vi "Datacluster_modify column.vi"(6 "tolerance":dbl=0.0005 format="%.3e", 7 "ascending":bool, 9 "Sort?":bool, 10 "Datasets to be processed":T3(array[cluster])=[{"String"="KR6_Rh3In3Ge4", "Boolean"=TRUE, "begin"=0, "length"=99, "y weight"=1.0}], 11 "data cluster":cluster{"all rows":dbl[][]}[](array[cluster])=[{"all rows"=[[292.0, 292.9164, 75.02219, 292.5198, 292.873, 0.08675399, 165.5123, 4.898979, 292.4821, 292.7706, 292.492, 292.5008, 293.2383, 292.873, 25.04327, 12.87815, 8.722502e-06, 147301.0, 0.0, 49.12202, 7.026817e-06], [292.0, 292.6799, 51.88008, 291.997, 292.6172, 0.1254523, 164.8345, 4.898979, 291.9992, 292.2308, 292.069, 291.9987, 292.9044, 292.6172, 16.68079, 8.502932, 7.87955e-06, 148972.5, 0.0, 52.73522, 7.82408e-06], [289.0, 289.5872, 53.36827, 288.998, 289.5262, 0.121954, 164.6135, 4.898979, 288.9966, 289.0375, 288.9818, 288.9977, 289.7039, 289.5262, 16.9019, 8.586199, 8.115929e-06, 149524.0, 0.0, 53.28857, 7.979706e-06], [286.0, 286.5259, 49.68945, 285.998, 286.4604, 0.130983, 164.4479, 4.898979, 285.9991, 285.8497, 285.9015, 285.9993, 286.5396, 286.4604, 16.3069, 8.351839, 7.550718e-06, 150070.2, 0.0, 49.26372, 7.019865e-06], [283.0, 283.4711, 53.72872, 283.0, 283.4105, 0.1211359, 164.3414, 4.898979, 282.9993, 282.7069, 282.8492, 283.0001, 283.3894, 283.4105, 16.49914, 8.324846, 8.321034e-06, 150632.6, 0.0, 53.01569, 7.9647e-06], [280.0, 280.4225, 55.74425, 280.001, 280.3641, 0.116756, 164.0834, 4.898979, 279.9989, 279.5874, 279.805, 279.9995, 280.2632, 280.3641, 16.65599, 8.355238, 8.692565e-06, 151182.8, 0.0, 57.0127, 8.356655e-06], [277.0, 277.4087, 53.59749, 277.0, 277.348, 0.1214324, 163.8697, 4.898979, 276.999, 276.4814, 276.7861, 277.0003, 277.1648, 277.348, 16.48811, 8.322479, 8.417088e-06, 151713.2, 0.0, 56.02918, 8.50766e-06], [274.0, 274.42, 54.6898, 274.001, 274.3605, 0.1190071, 163.7107, 4.898979, 273.9996, 273.4294, 273.7956, 274.0001, 274.1133, 274.3605, 16.45529, 8.266658, 8.774592e-06, 152257.0, 0.0, 55.53214, 8.58475e-06], [271.0, 271.4452, 55.7095, 271.001, 271.3868, 0.1168288, 163.585, 4.898979, 270.9994, 270.3922, 270.812, 270.9999, 271.0838, 271.3868, 16.27431, 8.125881, 8.904832e-06, 152814.4, 0.0, 56.2198, 8.635062e-06], [268.0, 268.4699, 56.23065, 268.001, 268.412, 0.115746, 163.4811, 4.898979, 267.9992, 267.3543, 267.8305, 267.9997, 268.0515, 268.412, 16.14259, 8.031859, 9.125312e-06, 153358.0, 0.0, 56.47631, 9.315139e-06], [265.0, 265.504, 56.7819, 265.0, 265.4467, 0.1146223, 163.391, 4.898979, 264.9995, 264.3426, 264.8619, 264.9997, 265.042, 265.4467, 16.08378, 7.981424, 9.334535e-06, 153898.2, 0.0, 56.33507, 9.071532e-06], [262.0, 262.5402, 56.3029, 261.999, 262.4824, 0.1155975, 163.3034, 4.898979, 261.9999, 261.3382, 261.8933, 262.0, 262.0429, 262.4824, 15.96119, 7.921869, 9.410211e-06, 154447.6, 0.0, 56.37045, 9.069828e-06], [259.0, 259.5962, 58.10709, 259.0, 259.5401, 0.1120083, 163.2193, 4.898979, 258.9994, 258.3609, 258.9463, 258.9997, 259.0668, 259.5401, 15.93857, 7.860623, 9.705625e-06, 154984.0, 0.0, 56.57644, 9.146704e-06], [256.0, 256.6687, 56.23365, 255.999, 256.6109, 0.1157399, 163.1493, 4.898979, 255.999, 255.398, 256.0085, 255.9989, 256.1162, 256.6109, 15.6581, 7.744409, 9.492895e-06, 155529.5, 0.0, 56.48109, 9.279682e-06], [253.0, 253.5733, 56.38813, 253.0, 253.53, 0.08656709, 163.0587, 4.242641, 252.9989, 252.4462, 253.0724, 252.9998, 252.9904, 253.53, 15.52846, 7.664103, 9.532705e-06, 156076.4, 0.0, 55.89689, 9.252784e-06], [250.0, 250.6412, 54.69462, 250.0, 250.5966, 0.08924747, 162.9786, 4.242641, 250.0002, 249.4823, 250.1305, 250.0004, 250.0376, 250.5966, 15.19496, 7.512066, 9.061377e-06, 156639.2, 0.0, 56.67262, 9.431853e-06], [247.0, 247.7008, 56.19418, 247.001, 247.6573, 0.08686587, 162.8957, 4.242641, 246.9987, 246.5324, 247.1849, 247.0003, 247.0917, 247.6573, 15.12285, 7.431846, 9.658179e-06, 157187.5, 0.0, 58.88652, 9.951588e-06], [244.0, 244.756, 57.27194, 243.999, 244.7134, 0.08523119, 162.8167, 4.242641, 243.9985, 243.5809, 244.2381, 243.9991, 244.1415, 244.7134, 15.06449, 7.372421, 1.015879e-05, 157736.6, 0.0, 57.34745, 9.89733e-06], [241.0, 241.8457, 56.35606, 240.999, 241.8024, 0.08661635, 162.7319, 4.242641, 240.9999, 240.6596, 241.3181, 240.9994, 241.2305, 241.8024, 14.76138, 7.218644, 1.001309e-05, 158281.2, 0.0, 55.59713, 9.467991e-06], [238.0, 238.9209, 56.78944, 238.0, 238.8779, 0.08595534, 162.6528, 4.242641, 237.9983, 237.7335, 238.3869, 237.9997, 238.3104, 238.8779, 14.65413, 7.147241, 9.925203e-06, 158821.8, 0.0, 57.4055, 9.991189e-06], [235.0, 235.8546, 58.50336, 235.0, 235.8233, 0.0625779, 162.5361, 3.674235, 234.9997, 234.8069, 235.452, 234.9992, 235.2407, 235.8233, 14.56547, 7.060409, 1.032292e-05, 159362.6, 0.0, 58.88609, 1.077016e-05], [232.0, 232.9135, 58.7887, 232.0, 232.8823, 0.06227416, 162.4497, 3.674235, 231.9992, 231.8697, 232.505, 232.0, 232.3093, 232.8823, 14.4148, 6.969601, 1.039831e-05, 159894.4, 0.0, 60.38943, 1.099243e-05], [229.0, 229.9683, 52.90027, 228.999, 229.9337, 0.06920602, 162.3651, 3.674235, 228.9996, 228.9262, 229.5497, 228.9995, 229.3795, 229.9337, 13.95679, 6.834046, 9.47672e-06, 160443.8, 0.0, 55.18934, 1.011709e-05], [226.0, 227.0314, 55.01033, 226.001, 226.9982, 0.06655145, 162.2802, 3.674235, 225.9986, 225.9999, 226.6072, 226.0003, 226.4574, 226.9982, 13.87658, 6.741458, 1.003314e-05, 160986.4, 0.0, 56.71966, 9.916942e-06], [223.0, 224.0942, 54.51703, 222.999, 224.0606, 0.06715364, 162.193, 3.674235, 222.9989, 223.0755, 223.6635, 222.999, 223.5397, 224.0606, 13.63051, 6.611919, 9.828761e-06, 161551.5, 0.0, 57.5095, 1.147469e-05], [220.0, 221.1488, 53.22712, 219.999, 221.1144, 0.06878105, 162.1079, 3.674235, 219.9987, 220.1357, 220.7061, 219.9996, 220.6128, 221.1144, 13.28219, 6.44084, 9.954398e-06, 162102.9, 0.0, 56.94044, 1.050179e-05], [217.0, 218.18, 55.6197, 217.0, 218.1471, 0.06582231, 162.0181, 3.674235, 216.9999, 217.1911, 217.7388, 216.9998, 217.6652, 218.1471, 13.33998, 6.426719, 1.030691e-05, 162650.0, 0.0, 54.95497, 1.056938e-05], [214.0, 215.2041, 52.74785, 214.001, 215.1694, 0.069406, 161.9245, 3.674235, 213.9993, 214.2305, 214.7574, 214.0001, 214.7119, 215.1694, 13.16094, 6.381908, 1.041787e-05, 163183.7, 0.0, 54.82949, 1.00501e-05], [211.0, 212.2438, 53.2594, 210.999, 212.2094, 0.06873936, 161.8459, 3.674235, 211.0002, 211.2871, 211.7895, 210.9995, 211.7758, 212.2094, 12.92852, 6.240668, 1.038931e-05, 163737.5, 0.0, 53.69054, 9.725446e-06], [208.0, 209.2728, 54.18705, 208.0, 209.239, 0.06756258, 161.7569, 3.674235, 207.9997, 208.341, 208.8189, 207.9994, 208.8287, 209.239, 12.96622, 6.244319, 1.030433e-05, 164296.5, 0.0, 51.99244, 9.937355e-06], [205.0, 206.3015, 47.85468, 204.999, 206.2633, 0.0765028, 161.669, 3.674235, 204.9996, 205.3777, 205.8335, 204.9997, 205.8839, 206.2633, 12.49721, 6.108157, 8.850608e-06, 164832.5, 0.0, 52.33099, 1.025279e-05], [202.0, 203.3115, 47.77909, 202.0, 203.2732, 0.07662382, 161.578, 3.674235, 201.9992, 202.4024, 202.836, 201.9998, 202.9163, 203.2732, 12.32563, 6.011273, 9.175306e-06, 165383.8, 0.0, 49.48042, 9.796374e-06], [199.0, 200.3016, 48.81196, 199.001, 200.2641, 0.07500245, 161.4837, 3.674235, 198.9994, 199.4091, 199.8188, 199.0009, 199.9294, 200.2641, 12.19196, 5.913105, 9.19541e-06, 165931.2, 0.0, 48.99235, 9.119814e-06], [196.0, 197.3124, 46.33101, 196.0, 197.2728, 0.07901871, 161.3904, 3.674235, 195.9999, 196.4343, 196.8208, 195.9996, 196.9654, 197.2728, 11.90443, 5.801792, 9.14851e-06, 166481.8, 0.0, 47.56836, 9.084771e-06], [193.0, 194.3294, 48.48906, 193.0, 194.2917, 0.07550192, 161.2938, 3.674235, 192.9996, 193.4505, 193.8166, 192.9997, 194.001, 194.2917, 11.49295, 5.526408, 9.320439e-06, 167039.8, 0.0, 49.01581, 9.34799e-06], [190.0, 191.3157, 47.75745, 189.999, 191.2773, 0.07665855, 161.2094, 3.674235, 190.0005, 190.4523, 190.7964, 189.9991, 191.0099, 191.2773, 11.31843, 5.442408, 9.51165e-06, 167586.2, 0.0, 47.72681, 9.290438e-06], [187.0, 188.2909, 46.66995, 186.998, 188.2517, 0.07844485, 161.1183, 3.674235, 186.9996, 187.4401, 187.7654, 187.0006, 188.0048, 188.2517, 11.22194, 5.408542, 9.210011e-06, 168125.0, 0.0, 47.7442, 9.335471e-06], [184.0, 185.2608, 45.59003, 184.0, 185.2207, 0.08030301, 161.02, 3.674235, 183.9996, 184.4185, 184.7246, 183.9997, 184.9949, 185.2207, 10.97692, 5.291597, 8.987941e-06, 168671.0, 0.0, 45.18603, 8.882518e-06], [181.0, 182.2488, 42.55964, 181.0, 182.2057, 0.08602087, 160.9233, 3.674235, 180.9996, 181.4114, 181.7032, 180.9994, 182.0001, 182.2057, 10.7433, 5.21988, 8.481294e-06, 169224.8, 0.0, 42.92117, 8.932989e-06], [178.0, 179.2327, 43.4817, 178.0, 179.1906, 0.08419672, 160.8244, 3.674235, 177.9992, 178.3866, 178.6756, 177.9989, 178.9857, 179.1906, 10.55317, 5.093926, 8.674955e-06, 169761.4, 0.0, 46.08075, 9.801831e-06], [175.0, 176.1988, 41.91763, 174.999, 176.1551, 0.08733836, 160.7272, 3.674235, 174.9992, 175.3492, 175.6323, 175.0005, 175.9594, 176.1551, 10.39018, 5.032765, 8.418331e-06, 170337.0, 0.0, 41.27729, 8.256854e-06], [172.0, 173.1462, 40.78401, 171.998, 173.1014, 0.08976599, 160.6309, 3.674235, 171.9994, 172.2934, 172.5681, 172.0007, 172.9165, 173.1014, 10.17369, 4.933174, 8.561175e-06, 170884.7, 0.0, 42.0311, 8.954053e-06], [169.0, 170.1156, 39.52542, 169.002, 170.0692, 0.09262438, 160.5319, 3.674235, 168.9985, 169.2597, 169.5281, 169.0004, 169.8935, 170.0692, 10.01111, 4.866947, 7.889127e-06, 171427.6, 0.0, 41.17875, 8.476864e-06], [166.0, 167.0848, 37.75683, 166.0, 167.0363, 0.09696304, 160.4351, 3.674235, 165.9992, 166.2177, 166.4835, 165.9991, 166.8676, 167.0363, 9.732579, 4.745978, 7.667965e-06, 171976.2, 0.0, 40.17138, 7.923543e-06], [163.0, 164.0348, 37.48756, 163.0, 163.986, 0.09765951, 160.3364, 3.674235, 162.9994, 163.1585, 163.4224, 162.9994, 163.8198, 163.986, 9.565177, 4.656068, 7.403833e-06, 172519.0, 0.0, 37.92251, 7.706918e-06], [160.0, 160.9789, 37.24322, 160.0, 160.9297, 0.09830023, 160.2345, 3.674235, 159.9997, 160.0851, 160.3523, 159.9997, 160.7607, 160.9297, 9.362346, 4.545693, 7.846706e-06, 173077.8, 0.0, 38.13007, 8.027448e-06], [157.0, 157.7978, 36.56221, 157.0, 157.7603, 0.07509838, 160.1422, 3.181981, 157.0001, 157.0355, 157.3161, 157.0001, 157.5547, 157.7603, 9.136679, 4.431653, 7.299468e-06, 173622.6, 0.0, 36.74182, 7.431135e-06], [154.0, 154.7562, 36.11287, 153.999, 154.7182, 0.0760328, 160.039, 3.181981, 154.0002, 153.9788, 154.2641, 153.9991, 154.5089, 154.7182, 8.931389, 4.324545, 7.829839e-06, 174165.6, 0.0, 37.11626, 7.907207e-06], [151.0, 151.7025, 35.56308, 151.001, 151.6639, 0.07720823, 159.94, 3.181981, 150.9997, 150.9063, 151.1997, 151.0003, 151.4478, 151.6639, 8.772177, 4.245581, 7.074522e-06, 174712.4, 0.0, 34.8322, 7.606191e-06], [148.0, 148.6425, 34.07633, 148.001, 148.6022, 0.08057683, 159.8368, 3.181981, 148.0007, 147.8203, 148.1272, 148.0007, 148.376, 148.6022, 8.538666, 4.143502, 7.012669e-06, 175270.5, 0.0, 35.5259, 7.773223e-06], [145.0, 145.6151, 32.94494, 145.0, 145.5734, 0.08334398, 159.7329, 3.181981, 144.9995, 144.7711, 145.0917, 145.0, 145.3362, 145.5734, 8.402115, 4.089585, 6.717016e-06, 175825.6, 0.0, 34.5873, 7.462285e-06], [142.0, 142.4503, 32.69128, 141.998, 142.4188, 0.062993, 159.6235, 2.755676, 141.9999, 141.7087, 142.045, 141.998, 142.1454, 142.4188, 8.112161, 3.93007, 6.970786e-06, 176365.9, 0.0, 33.20516, 7.879391e-06], [139.0, 139.3994, 31.76623, 139.001, 139.367, 0.06482741, 159.5169, 2.755676, 138.9981, 138.6308, 138.9849, 138.9994, 139.0777, 139.367, 7.985541, 3.877216, 6.982463e-06, 176903.8, 0.0, 32.45839, 6.596733e-06], [136.0, 136.3652, 31.01851, 135.998, 136.332, 0.0663901, 159.4101, 2.755676, 135.9989, 135.5674, 135.9417, 135.999, 136.0241, 136.332, 7.79429, 3.784086, 6.795836e-06, 177452.3, 0.0, 32.19581, 6.462182e-06], [133.0, 133.3502, 30.5601, 133.0, 133.3165, 0.06738596, 159.3015, 2.755676, 132.9992, 132.5206, 132.9147, 132.9999, 132.9898, 133.3165, 7.59515, 3.680558, 6.903421e-06, 178000.4, 0.0, 31.58324, 6.744551e-06], [130.0, 130.2115, 29.16558, 130.0, 130.185, 0.05295598, 159.122, 2.386485, 130.0005, 129.4585, 129.875, 129.9997, 129.8214, 130.185, 7.33831, 3.563506, 7.084772e-06, 178528.9, 0.0, 30.31422, 6.637657e-06], [127.0, 127.0902, 28.66261, 127.0, 127.07, 0.04041393, 159.0379, 2.066757, 126.9998, 126.3926, 126.8334, 126.9993, 126.6696, 127.07, 7.211448, 3.501876, 6.550803e-06, 179072.6, 0.0, 27.84635, 6.955272e-06], [124.0, 124.092, 28.58992, 124.0, 124.0717, 0.04051669, 158.9287, 2.066757, 124.0006, 123.3645, 123.8279, 123.9994, 123.6488, 124.0717, 7.012868, 3.390962, 7.173261e-06, 179624.9, 0.0, 28.22442, 4.92486e-06], [121.0, 121.0173, 26.81918, 120.999, 121.0011, 0.03239384, 158.8124, 1.789864, 120.9991, 120.3247, 120.8123, 120.9995, 120.5459, 121.0011, 6.797255, 3.304885, 4.45575e-06, 180140.8, 0.0, 29.19013, 5.915953e-06], [118.0, 117.9932, 25.80576, 117.999, 117.9764, 0.03366599, 158.6989, 1.789864, 117.9995, 117.2703, 117.781, 118.0, 117.4994, 117.9764, 6.568201, 3.195852, 5.482144e-06, 180683.1, 0.0, 27.08986, 6.913137e-06], [115.0, 115.0141, 25.65538, 114.998, 114.9971, 0.03386332, 158.5865, 1.789864, 115.0005, 114.2643, 114.7982, 114.9996, 114.497, 114.9971, 6.423356, 3.116589, 5.528924e-06, 181217.8, 0.0, 26.62919, 5.253105e-06], [112.0, 112.0203, 26.59349, 112.001, 112.004, 0.03266877, 158.4708, 1.789864, 111.9995, 111.2424, 111.7992, 111.9994, 111.4798, 112.004, 6.320665, 3.040642, 5.840544e-06, 181744.4, 0.0, 26.32533, 6.485414e-06], [109.0, 109.016, 25.89338, 109.0, 108.9992, 0.03355207, 158.3582, 1.789864, 109.0002, 108.2095, 108.7884, 108.9998, 108.4539, 108.9992, 6.13315, 2.948822, 4.976681e-06, 182293.6, 0.0, 25.56833, 6.586255e-06], [106.0, 106.0601, 24.74948, 105.999, 106.0426, 0.03510282, 158.2417, 1.789864, 106.0009, 105.2233, 105.8221, 105.9986, 105.4789, 106.0426, 5.82098, 2.795607, 5.520496e-06, 182820.9, 0.0, 25.1926, 5.082759e-06], [103.0, 103.1012, 23.47957, 102.999, 103.0827, 0.03700138, 158.1265, 1.789864, 102.9994, 102.2249, 102.852, 102.9995, 102.4926, 103.0827, 5.610787, 2.701479, 5.748678e-06, 183358.4, 0.0, 24.56658, 4.990891e-06], [100.0, 100.1194, 24.40213, 100.0, 100.1016, 0.03560248, 158.0093, 1.789864, 99.99963, 99.21942, 99.86005, 99.99973, 99.49659, 100.1016, 5.418124, 2.579388, 5.193695e-06, 183898.6, 0.0, 24.73305, 4.828259e-06], [97.0, 97.17382, 23.39176, 97.0015, 97.15525, 0.03714027, 157.8955, 1.789864, 96.99884, 96.25454, 96.90598, 96.99946, 96.54095, 97.15525, 5.252876, 2.504921, 5.62191e-06, 184439.7, 0.0, 23.73066, 5.229691e-06], [94.0, 94.20774, 23.22087, 94.0002, 94.18903, 0.0374136, 157.7782, 1.789864, 93.99808, 93.27039, 93.92858, 94.00004, 93.56826, 94.18903, 5.073145, 2.409457, 5.538685e-06, 184984.4, 0.0, 23.61211, 6.687232e-06], [91.0, 91.13359, 22.59694, 91.0003, 91.11917, 0.02883498, 157.6522, 1.550068, 91.0004, 90.31659, 90.91559, 90.9996, 90.54901, 91.11917, 4.827745, 2.285596, 4.255465e-06, 185533.6, 0.0, 21.92768, 5.296259e-06], [88.0, 88.18123, 22.48137, 87.9991, 88.16674, 0.02898322, 157.5325, 1.550068, 87.9996, 87.35154, 87.95371, 87.99927, 87.59355, 88.16674, 4.645815, 2.189353, 4.903361e-06, 186084.2, 0.0, 21.34062, 6.20428e-06], [85.0, 85.24232, 22.00163, 84.9979, 85.22751, 0.02961518, 157.4127, 1.550068, 85.00029, 84.40605, 85.0051, 84.99872, 84.65807, 85.22751, 4.439868, 2.085645, 3.898806e-06, 186641.8, 0.0, 20.03455, 4.048067e-06], [82.0, 82.2906, 20.26436, 82.0003, 82.27452, 0.0321541, 157.2935, 1.550068, 81.99943, 81.3944, 82.04882, 81.99944, 81.65225, 82.27452, 4.366601, 2.069786, 4.384861e-06, 187170.4, 0.0, 19.93068, 5.169709e-06], [79.0, 79.35992, 20.65986, 78.9998, 79.34415, 0.03153857, 157.175, 1.550068, 78.99976, 78.46501, 79.10271, 78.99972, 78.73799, 79.34415, 4.123809, 1.934396, 5.660535e-06, 187707.0, 0.0, 20.24228, 3.521332e-06], [76.0, 76.34799, 18.14755, 76.0001, 76.33453, 0.02692852, 157.0442, 1.342398, 75.9988, 75.52364, 76.14176, 76.00082, 75.74333, 76.33453, 3.879228, 1.836679, 5.277406e-06, 188227.8, 0.0, 18.3202, 4.280038e-06], [73.0, 73.40674, 18.83722, 72.9989, 73.39377, 0.02594261, 156.9286, 1.342398, 72.9991, 72.60294, 73.19315, 72.99918, 72.82951, 73.39377, 3.728216, 1.746902, 4.133453e-06, 188764.6, 0.0, 20.32012, 4.874801e-06], [70.0, 70.45695, 17.51673, 70.0003, 70.443, 0.02789829, 156.8115, 1.342398, 70.00086, 69.67221, 70.23128, 69.99956, 69.91183, 70.443, 3.505012, 1.644658, 3.415282e-06, 189312.8, 0.0, 18.10538, 3.636672e-06], [67.0, 67.51137, 17.06142, 66.9986, 67.49705, 0.0286428, 156.6926, 1.342398, 67.0003, 66.75251, 67.27265, 66.99976, 67.00556, 67.49705, 3.329935, 1.557489, 3.637388e-06, 189850.0, 0.0, 17.81273, 2.997229e-06], [64.0, 64.55299, 16.05667, 63.9994, 64.53777, 0.03043512, 156.572, 1.342398, 63.99965, 63.82388, 64.3001, 64.00019, 64.09199, 64.53777, 3.155975, 1.477454, 3.836114e-06, 190372.4, 0.0, 16.65761, 3.137167e-06], [61.0, 61.59684, 15.15327, 61.0012, 61.58071, 0.03224959, 156.4552, 1.342398, 61.00003, 60.89696, 61.32582, 60.99921, 61.18411, 61.58071, 2.932403, 1.370073, 2.715446e-06, 190890.4, 0.0, 15.46223, 4.794554e-06], [58.0, 58.6279, 14.0184, 58.0008, 58.61047, 0.03486038, 156.3434, 1.342398, 57.99915, 57.96364, 58.33762, 57.99934, 58.27135, 58.61047, 2.745862, 1.284894, 2.94282e-06, 191408.4, 0.0, 14.4151, 4.772166e-06], [55.0, 55.65962, 12.33515, 55.0029, 55.63981, 0.03961743, 156.2312, 1.342398, 54.99762, 55.02696, 55.34105, 55.0008, 55.36534, 55.63981, 2.519189, 1.185287, 3.164869e-06, 191919.5, 0.0, 12.86659, 1.828514e-06], [52.0, 52.69421, 11.21244, 51.999, 52.67242, 0.04358434, 156.12, 1.342398, 51.99888, 52.0955, 52.34609, 51.99949, 52.46542, 52.67242, 2.286444, 1.075562, 2.081657e-06, 192439.7, 0.0, 11.76603, 2.789106e-06], [49.0, 49.61418, 9.645293, 49.001, 49.59518, 0.03799937, 156.0042, 1.162551, 48.99919, 49.13845, 49.32293, 49.00038, 49.4487, 49.59518, 2.049105, 0.9693383, 2.419945e-06, 192925.6, 0.0, 10.21014, 2.551699e-06], [46.0, 46.64398, 8.849838, 46.0014, 46.62327, 0.04141489, 155.8991, 1.162551, 45.99971, 46.20159, 46.31906, 45.99925, 46.54721, 46.62327, 1.829977, 0.8624549, 2.062263e-06, 193484.8, 0.0, 8.642792, 8.766135e-07], [43.0, 43.63805, 8.111564, 43.0, 43.61546, 0.04518427, 155.7963, 1.162551, 43.00087, 43.23263, 43.28277, 42.99939, 43.6105, 43.61546, 1.669476, 0.7863123, 2.202847e-06, 194031.9, 0.0, 8.304894, 2.187056e-06], [40.0, 40.60721, 7.850611, 39.9976, 40.58387, 0.04668618, 155.6928, 1.162551, 39.99903, 40.24392, 40.22946, 39.99922, 40.64502, 40.58387, 1.579687, 0.7417823, 1.934699e-06, 194511.3, 0.0, 7.823251, 1.052641e-06], [37.0, 37.55588, 7.570818, 37.0021, 37.53168, 0.04841156, 155.5887, 1.162551, 36.99997, 37.23081, 37.15568, 36.99985, 37.65521, 37.53168, 1.491856, 0.6986331, 1.616464e-06, 195029.6, 0.0, 7.701154, 1.426829e-06], [34.0, 34.39013, 7.129456, 34.002, 34.37085, 0.03855642, 155.4653, 1.006799, 34.00288, 34.19961, 34.07078, 33.99971, 34.53824, 34.37085, 1.389701, 0.6498903, 1.456064e-06, 195501.9, 0.0, 7.197325, 1.830936e-06], [31.0, 31.3295, 6.959681, 30.9971, 31.30975, 0.03949697, 155.3693, 1.006799, 31.00027, 31.15947, 30.98673, 30.99905, 31.52198, 31.30975, 1.305866, 0.6077944, 1.746532e-06, 195974.6, 0.0, 6.855044, 1.3535e-07], [28.0, 28.257, 6.444445, 28.0083, 28.23568, 0.04265477, 155.2754, 1.006799, 27.99751, 28.08427, 27.88122, 28.00025, 28.48138, 28.23568, 1.20443, 0.5603139, 1.207888e-06, 196438.7, 0.0, 6.465166, 2.29124e-06], [25.0, 25.1858, 5.908139, 25.0055, 25.16253, 0.04652672, 155.1906, 1.006799, 25.00147, 24.99086, 24.77406, 24.99832, 25.42586, 25.16253, 1.084087, 0.5032175, 9.614257e-07, 196931.6, 0.0, 5.92471, -5.51895e-08], [22.0, 22.16916, 5.305623, 21.9854, 22.14325, 0.05181037, 155.1142, 1.006799, 22.00671, 21.91764, 21.70696, 21.99982, 22.40575, 22.14325, 0.959603, 0.4446781, 7.916026e-07, 197380.4, 0.0, 5.277611, 2.768679e-07], [19.0, 19.30572, 4.637635, 18.9844, 19.27608, 0.05927295, 155.0499, 1.006799, 18.99661, 18.95241, 18.76765, 19.00061, 19.52011, 19.27608, 0.8426237, 0.390679, 5.587576e-07, 197860.4, 0.0, 4.670142, -7.621961e-08], [16.0, 16.50024, 3.972702, 16.0034, 16.46565, 0.06919378, 154.9962, 1.006799, 15.99681, 16.00464, 15.86607, 15.99389, 16.67341, 16.46565, 0.7071578, 0.3270905, 3.955843e-07, 198345.2, 0.0, 3.981336, -9.093087e-09], [13.0, 13.71888, 3.255681, 13.0265, 13.67666, 0.08443282, 154.9529, 1.006799, 12.99021, 12.98951, 12.9155, 12.99523, 13.83511, 13.67666, 0.5650661, 0.2606204, 4.899574e-08, 199058.5, 0.0, 3.267024, -3.089664e-07], [10.0, 11.02144, 2.634719, 9.9178, 10.96927, 0.1043323, 154.9244, 1.006799, 9.979209, 9.944225, 9.937939, 9.981572, 11.07989, 10.96927, 0.4191188, 0.1915213, 3.509129e-08, 199788.6, 0.0, 2.637912, 3.892924e-07], [7.0, 8.207977, 2.280254, 7.0263, 8.162771, 0.09041306, 154.877, 0.8719131, 6.996675, 6.899136, 6.944581, 6.995916, 8.207738, 8.162771, 0.272072, 0.1212537, 1.590448e-07, 200474.8, 0.0, 2.226699, -2.06841e-07], [4.0, 6.17061, 6.914511, 3.9852, 6.155702, 0.02981624, 154.8519, 0.8719131, 4.007358, 3.946248, 3.912001, 4.007225, 6.219766, 6.155702, 0.1566822, 0.06587024, 3.496313e-07, 201190.7, 0.0, 6.388795, -3.268214e-08], [2.0, 3.439481, -0.8426919, 2.2818, 3.470062, -0.06116255, 154.8119, 0.4359565, 2.275721, 2.314741, 2.136495, 2.275818, 3.587147, 3.470062, 0.06999886, 0.02771, -3.623877e-09, 201712.2, 0.0, -0.8426919, -3.623877e-09]]}]) -> (3 "data cluster out":cluster{"all rows":dbl[][]}[](array[cluster])=[{"all rows"=[[292.0, 292.9164, 75.02219, 292.5198, 292.873, 0.08675399, 165.5123, 4.898979, 292.4821, 292.7706, 292.492, 292.5008, 293.2383, 292.873, 25.04327, 12.87815, 8.722502e-06, 147301.0, 0.0, 49.12202, 7.026817e-06], [292.0, 292.6799, 51.88008, 291.997, 292.6172, 0.1254523, 164.8345, 4.898979, 291.9992, 292.2308, 292.069, 291.9987, 292.9044, 292.6172, 16.68079, 8.502932, 7.87955e-06, 148972.5, 0.0, 52.73522, 7.82408e-06], [289.0, 289.5872, 53.36827, 288.998, 289.5262, 0.121954, 164.6135, 4.898979, 288.9966, 289.0375, 288.9818, 288.9977, 289.7039, 289.5262, 16.9019, 8.586199, 8.115929e-06, 149524.0, 0.0, 53.28857, 7.979706e-06], [286.0, 286.5259, 49.68945, 285.998, 286.4604, 0.130983, 164.4479, 4.898979, 285.9991, 285.8497, 285.9015, 285.9993, 286.5396, 286.4604, 16.3069, 8.351839, 7.550718e-06, 150070.2, 0.0, 49.26372, 7.019865e-06], [283.0, 283.4711, 53.72872, 283.0, 283.4105, 0.1211359, 164.3414, 4.898979, 282.9993, 282.7069, 282.8492, 283.0001, 283.3894, 283.4105, 16.49914, 8.324846, 8.321034e-06, 150632.6, 0.0, 53.01569, 7.9647e-06], [280.0, 280.4225, 55.74425, 280.001, 280.3641, 0.116756, 164.0834, 4.898979, 279.9989, 279.5874, 279.805, 279.9995, 280.2632, 280.3641, 16.65599, 8.355238, 8.692565e-06, 151182.8, 0.0, 57.0127, 8.356655e-06], [277.0, 277.4087, 53.59749, 277.0, 277.348, 0.1214324, 163.8697, 4.898979, 276.999, 276.4814, 276.7861, 277.0003, 277.1648, 277.348, 16.48811, 8.322479, 8.417088e-06, 151713.2, 0.0, 56.02918, 8.50766e-06], [274.0, 274.42, 54.6898, 274.001, 274.3605, 0.1190071, 163.7107, 4.898979, 273.9996, 273.4294, 273.7956, 274.0001, 274.1133, 274.3605, 16.45529, 8.266658, 8.774592e-06, 152257.0, 0.0, 55.53214, 8.58475e-06], [271.0, 271.4452, 55.7095, 271.001, 271.3868, 0.1168288, 163.585, 4.898979, 270.9994, 270.3922, 270.812, 270.9999, 271.0838, 271.3868, 16.27431, 8.125881, 8.904832e-06, 152814.4, 0.0, 56.2198, 8.635062e-06], [268.0, 268.4699, 56.23065, 268.001, 268.412, 0.115746, 163.4811, 4.898979, 267.9992, 267.3543, 267.8305, 267.9997, 268.0515, 268.412, 16.14259, 8.031859, 9.125312e-06, 153358.0, 0.0, 56.47631, 9.315139e-06], [265.0, 265.504, 56.7819, 265.0, 265.4467, 0.1146223, 163.391, 4.898979, 264.9995, 264.3426, 264.8619, 264.9997, 265.042, 265.4467, 16.08378, 7.981424, 9.334535e-06, 153898.2, 0.0, 56.33507, 9.071532e-06], [262.0, 262.5402, 56.3029, 261.999, 262.4824, 0.1155975, 163.3034, 4.898979, 261.9999, 261.3382, 261.8933, 262.0, 262.0429, 262.4824, 15.96119, 7.921869, 9.410211e-06, 154447.6, 0.0, 56.37045, 9.069828e-06], [259.0, 259.5962, 58.10709, 259.0, 259.5401, 0.1120083, 163.2193, 4.898979, 258.9994, 258.3609, 258.9463, 258.9997, 259.0668, 259.5401, 15.93857, 7.860623, 9.705625e-06, 154984.0, 0.0, 56.57644, 9.146704e-06], [256.0, 256.6687, 56.23365, 255.999, 256.6109, 0.1157399, 163.1493, 4.898979, 255.999, 255.398, 256.0085, 255.9989, 256.1162, 256.6109, 15.6581, 7.744409, 9.492895e-06, 155529.5, 0.0, 56.48109, 9.279682e-06], [253.0, 253.5733, 56.38813, 253.0, 253.53, 0.08656709, 163.0587, 4.242641, 252.9989, 252.4462, 253.0724, 252.9998, 252.9904, 253.53, 15.52846, 7.664103, 9.532705e-06, 156076.4, 0.0, 55.89689, 9.252784e-06], [250.0, 250.6412, 54.69462, 250.0, 250.5966, 0.08924747, 162.9786, 4.242641, 250.0002, 249.4823, 250.1305, 250.0004, 250.0376, 250.5966, 15.19496, 7.512066, 9.061377e-06, 156639.2, 0.0, 56.67262, 9.431853e-06], [247.0, 247.7008, 56.19418, 247.001, 247.6573, 0.08686587, 162.8957, 4.242641, 246.9987, 246.5324, 247.1849, 247.0003, 247.0917, 247.6573, 15.12285, 7.431846, 9.658179e-06, 157187.5, 0.0, 58.88652, 9.951588e-06], [244.0, 244.756, 57.27194, 243.999, 244.7134, 0.08523119, 162.8167, 4.242641, 243.9985, 243.5809, 244.2381, 243.9991, 244.1415, 244.7134, 15.06449, 7.372421, 1.015879e-05, 157736.6, 0.0, 57.34745, 9.89733e-06], [241.0, 241.8457, 56.35606, 240.999, 241.8024, 0.08661635, 162.7319, 4.242641, 240.9999, 240.6596, 241.3181, 240.9994, 241.2305, 241.8024, 14.76138, 7.218644, 1.001309e-05, 158281.2, 0.0, 55.59713, 9.467991e-06], [238.0, 238.9209, 56.78944, 238.0, 238.8779, 0.08595534, 162.6528, 4.242641, 237.9983, 237.7335, 238.3869, 237.9997, 238.3104, 238.8779, 14.65413, 7.147241, 9.925203e-06, 158821.8, 0.0, 57.4055, 9.991189e-06], [235.0, 235.8546, 58.50336, 235.0, 235.8233, 0.0625779, 162.5361, 3.674235, 234.9997, 234.8069, 235.452, 234.9992, 235.2407, 235.8233, 14.56547, 7.060409, 1.032292e-05, 159362.6, 0.0, 58.88609, 1.077016e-05], [232.0, 232.9135, 58.7887, 232.0, 232.8823, 0.06227416, 162.4497, 3.674235, 231.9992, 231.8697, 232.505, 232.0, 232.3093, 232.8823, 14.4148, 6.969601, 1.039831e-05, 159894.4, 0.0, 60.38943, 1.099243e-05], [229.0, 229.9683, 52.90027, 228.999, 229.9337, 0.06920602, 162.3651, 3.674235, 228.9996, 228.9262, 229.5497, 228.9995, 229.3795, 229.9337, 13.95679, 6.834046, 9.47672e-06, 160443.8, 0.0, 55.18934, 1.011709e-05], [226.0, 227.0314, 55.01033, 226.001, 226.9982, 0.06655145, 162.2802, 3.674235, 225.9986, 225.9999, 226.6072, 226.0003, 226.4574, 226.9982, 13.87658, 6.741458, 1.003314e-05, 160986.4, 0.0, 56.71966, 9.916942e-06], [223.0, 224.0942, 54.51703, 222.999, 224.0606, 0.06715364, 162.193, 3.674235, 222.9989, 223.0755, 223.6635, 222.999, 223.5397, 224.0606, 13.63051, 6.611919, 9.828761e-06, 161551.5, 0.0, 57.5095, 1.147469e-05], [220.0, 221.1488, 53.22712, 219.999, 221.1144, 0.06878105, 162.1079, 3.674235, 219.9987, 220.1357, 220.7061, 219.9996, 220.6128, 221.1144, 13.28219, 6.44084, 9.954398e-06, 162102.9, 0.0, 56.94044, 1.050179e-05], [217.0, 218.18, 55.6197, 217.0, 218.1471, 0.06582231, 162.0181, 3.674235, 216.9999, 217.1911, 217.7388, 216.9998, 217.6652, 218.1471, 13.33998, 6.426719, 1.030691e-05, 162650.0, 0.0, 54.95497, 1.056938e-05], [214.0, 215.2041, 52.74785, 214.001, 215.1694, 0.069406, 161.9245, 3.674235, 213.9993, 214.2305, 214.7574, 214.0001, 214.7119, 215.1694, 13.16094, 6.381908, 1.041787e-05, 163183.7, 0.0, 54.82949, 1.00501e-05], [211.0, 212.2438, 53.2594, 210.999, 212.2094, 0.06873936, 161.8459, 3.674235, 211.0002, 211.2871, 211.7895, 210.9995, 211.7758, 212.2094, 12.92852, 6.240668, 1.038931e-05, 163737.5, 0.0, 53.69054, 9.725446e-06], [208.0, 209.2728, 54.18705, 208.0, 209.239, 0.06756258, 161.7569, 3.674235, 207.9997, 208.341, 208.8189, 207.9994, 208.8287, 209.239, 12.96622, 6.244319, 1.030433e-05, 164296.5, 0.0, 51.99244, 9.937355e-06], [205.0, 206.3015, 47.85468, 204.999, 206.2633, 0.0765028, 161.669, 3.674235, 204.9996, 205.3777, 205.8335, 204.9997, 205.8839, 206.2633, 12.49721, 6.108157, 8.850608e-06, 164832.5, 0.0, 52.33099, 1.025279e-05], [202.0, 203.3115, 47.77909, 202.0, 203.2732, 0.07662382, 161.578, 3.674235, 201.9992, 202.4024, 202.836, 201.9998, 202.9163, 203.2732, 12.32563, 6.011273, 9.175306e-06, 165383.8, 0.0, 49.48042, 9.796374e-06], [199.0, 200.3016, 48.81196, 199.001, 200.2641, 0.07500245, 161.4837, 3.674235, 198.9994, 199.4091, 199.8188, 199.0009, 199.9294, 200.2641, 12.19196, 5.913105, 9.19541e-06, 165931.2, 0.0, 48.99235, 9.119814e-06], [196.0, 197.3124, 46.33101, 196.0, 197.2728, 0.07901871, 161.3904, 3.674235, 195.9999, 196.4343, 196.8208, 195.9996, 196.9654, 197.2728, 11.90443, 5.801792, 9.14851e-06, 166481.8, 0.0, 47.56836, 9.084771e-06], [193.0, 194.3294, 48.48906, 193.0, 194.2917, 0.07550192, 161.2938, 3.674235, 192.9996, 193.4505, 193.8166, 192.9997, 194.001, 194.2917, 11.49295, 5.526408, 9.320439e-06, 167039.8, 0.0, 49.01581, 9.34799e-06], [190.0, 191.3157, 47.75745, 189.999, 191.2773, 0.07665855, 161.2094, 3.674235, 190.0005, 190.4523, 190.7964, 189.9991, 191.0099, 191.2773, 11.31843, 5.442408, 9.51165e-06, 167586.2, 0.0, 47.72681, 9.290438e-06], [187.0, 188.2909, 46.66995, 186.998, 188.2517, 0.07844485, 161.1183, 3.674235, 186.9996, 187.4401, 187.7654, 187.0006, 188.0048, 188.2517, 11.22194, 5.408542, 9.210011e-06, 168125.0, 0.0, 47.7442, 9.335471e-06], [184.0, 185.2608, 45.59003, 184.0, 185.2207, 0.08030301, 161.02, 3.674235, 183.9996, 184.4185, 184.7246, 183.9997, 184.9949, 185.2207, 10.97692, 5.291597, 8.987941e-06, 168671.0, 0.0, 45.18603, 8.882518e-06], [181.0, 182.2488, 42.55964, 181.0, 182.2057, 0.08602087, 160.9233, 3.674235, 180.9996, 181.4114, 181.7032, 180.9994, 182.0001, 182.2057, 10.7433, 5.21988, 8.481294e-06, 169224.8, 0.0, 42.92117, 8.932989e-06], [178.0, 179.2327, 43.4817, 178.0, 179.1906, 0.08419672, 160.8244, 3.674235, 177.9992, 178.3866, 178.6756, 177.9989, 178.9857, 179.1906, 10.55317, 5.093926, 8.674955e-06, 169761.4, 0.0, 46.08075, 9.801831e-06], [175.0, 176.1988, 41.91763, 174.999, 176.1551, 0.08733836, 160.7272, 3.674235, 174.9992, 175.3492, 175.6323, 175.0005, 175.9594, 176.1551, 10.39018, 5.032765, 8.418331e-06, 170337.0, 0.0, 41.27729, 8.256854e-06], [172.0, 173.1462, 40.78401, 171.998, 173.1014, 0.08976599, 160.6309, 3.674235, 171.9994, 172.2934, 172.5681, 172.0007, 172.9165, 173.1014, 10.17369, 4.933174, 8.561175e-06, 170884.7, 0.0, 42.0311, 8.954053e-06], [169.0, 170.1156, 39.52542, 169.002, 170.0692, 0.09262438, 160.5319, 3.674235, 168.9985, 169.2597, 169.5281, 169.0004, 169.8935, 170.0692, 10.01111, 4.866947, 7.889127e-06, 171427.6, 0.0, 41.17875, 8.476864e-06], [166.0, 167.0848, 37.75683, 166.0, 167.0363, 0.09696304, 160.4351, 3.674235, 165.9992, 166.2177, 166.4835, 165.9991, 166.8676, 167.0363, 9.732579, 4.745978, 7.667965e-06, 171976.2, 0.0, 40.17138, 7.923543e-06], [163.0, 164.0348, 37.48756, 163.0, 163.986, 0.09765951, 160.3364, 3.674235, 162.9994, 163.1585, 163.4224, 162.9994, 163.8198, 163.986, 9.565177, 4.656068, 7.403833e-06, 172519.0, 0.0, 37.92251, 7.706918e-06], [160.0, 160.9789, 37.24322, 160.0, 160.9297, 0.09830023, 160.2345, 3.674235, 159.9997, 160.0851, 160.3523, 159.9997, 160.7607, 160.9297, 9.362346, 4.545693, 7.846706e-06, 173077.8, 0.0, 38.13007, 8.027448e-06], [157.0, 157.7978, 36.56221, 157.0, 157.7603, 0.07509838, 160.1422, 3.181981, 157.0001, 157.0355, 157.3161, 157.0001, 157.5547, 157.7603, 9.136679, 4.431653, 7.299468e-06, 173622.6, 0.0, 36.74182, 7.431135e-06], [154.0, 154.7562, 36.11287, 153.999, 154.7182, 0.0760328, 160.039, 3.181981, 154.0002, 153.9788, 154.2641, 153.9991, 154.5089, 154.7182, 8.931389, 4.324545, 7.829839e-06, 174165.6, 0.0, 37.11626, 7.907207e-06], [151.0, 151.7025, 35.56308, 151.001, 151.6639, 0.07720823, 159.94, 3.181981, 150.9997, 150.9063, 151.1997, 151.0003, 151.4478, 151.6639, 8.772177, 4.245581, 7.074522e-06, 174712.4, 0.0, 34.8322, 7.606191e-06], [148.0, 148.6425, 34.07633, 148.001, 148.6022, 0.08057683, 159.8368, 3.181981, 148.0007, 147.8203, 148.1272, 148.0007, 148.376, 148.6022, 8.538666, 4.143502, 7.012669e-06, 175270.5, 0.0, 35.5259, 7.773223e-06], [145.0, 145.6151, 32.94494, 145.0, 145.5734, 0.08334398, 159.7329, 3.181981, 144.9995, 144.7711, 145.0917, 145.0, 145.3362, 145.5734, 8.402115, 4.089585, 6.717016e-06, 175825.6, 0.0, 34.5873, 7.462285e-06], [142.0, 142.4503, 32.69128, 141.998, 142.4188, 0.062993, 159.6235, 2.755676, 141.9999, 141.7087, 142.045, 141.998, 142.1454, 142.4188, 8.112161, 3.93007, 6.970786e-06, 176365.9, 0.0, 33.20516, 7.879391e-06], [139.0, 139.3994, 31.76623, 139.001, 139.367, 0.06482741, 159.5169, 2.755676, 138.9981, 138.6308, 138.9849, 138.9994, 139.0777, 139.367, 7.985541, 3.877216, 6.982463e-06, 176903.8, 0.0, 32.45839, 6.596733e-06], [136.0, 136.3652, 31.01851, 135.998, 136.332, 0.0663901, 159.4101, 2.755676, 135.9989, 135.5674, 135.9417, 135.999, 136.0241, 136.332, 7.79429, 3.784086, 6.795836e-06, 177452.3, 0.0, 32.19581, 6.462182e-06], [133.0, 133.3502, 30.5601, 133.0, 133.3165, 0.06738596, 159.3015, 2.755676, 132.9992, 132.5206, 132.9147, 132.9999, 132.9898, 133.3165, 7.59515, 3.680558, 6.903421e-06, 178000.4, 0.0, 31.58324, 6.744551e-06], [130.0, 130.2115, 29.16558, 130.0, 130.185, 0.05295598, 159.122, 2.386485, 130.0005, 129.4585, 129.875, 129.9997, 129.8214, 130.185, 7.33831, 3.563506, 7.084772e-06, 178528.9, 0.0, 30.31422, 6.637657e-06], [127.0, 127.0902, 28.66261, 127.0, 127.07, 0.04041393, 159.0379, 2.066757, 126.9998, 126.3926, 126.8334, 126.9993, 126.6696, 127.07, 7.211448, 3.501876, 6.550803e-06, 179072.6, 0.0, 27.84635, 6.955272e-06], [124.0, 124.092, 28.58992, 124.0, 124.0717, 0.04051669, 158.9287, 2.066757, 124.0006, 123.3645, 123.8279, 123.9994, 123.6488, 124.0717, 7.012868, 3.390962, 7.173261e-06, 179624.9, 0.0, 28.22442, 4.92486e-06], [121.0, 121.0173, 26.81918, 120.999, 121.0011, 0.03239384, 158.8124, 1.789864, 120.9991, 120.3247, 120.8123, 120.9995, 120.5459, 121.0011, 6.797255, 3.304885, 4.45575e-06, 180140.8, 0.0, 29.19013, 5.915953e-06], [118.0, 117.9932, 25.80576, 117.999, 117.9764, 0.03366599, 158.6989, 1.789864, 117.9995, 117.2703, 117.781, 118.0, 117.4994, 117.9764, 6.568201, 3.195852, 5.482144e-06, 180683.1, 0.0, 27.08986, 6.913137e-06], [115.0, 115.0141, 25.65538, 114.998, 114.9971, 0.03386332, 158.5865, 1.789864, 115.0005, 114.2643, 114.7982, 114.9996, 114.497, 114.9971, 6.423356, 3.116589, 5.528924e-06, 181217.8, 0.0, 26.62919, 5.253105e-06], [112.0, 112.0203, 26.59349, 112.001, 112.004, 0.03266877, 158.4708, 1.789864, 111.9995, 111.2424, 111.7992, 111.9994, 111.4798, 112.004, 6.320665, 3.040642, 5.840544e-06, 181744.4, 0.0, 26.32533, 6.485414e-06], [109.0, 109.016, 25.89338, 109.0, 108.9992, 0.03355207, 158.3582, 1.789864, 109.0002, 108.2095, 108.7884, 108.9998, 108.4539, 108.9992, 6.13315, 2.948822, 4.976681e-06, 182293.6, 0.0, 25.56833, 6.586255e-06], [106.0, 106.0601, 24.74948, 105.999, 106.0426, 0.03510282, 158.2417, 1.789864, 106.0009, 105.2233, 105.8221, 105.9986, 105.4789, 106.0426, 5.82098, 2.795607, 5.520496e-06, 182820.9, 0.0, 25.1926, 5.082759e-06], [103.0, 103.1012, 23.47957, 102.999, 103.0827, 0.03700138, 158.1265, 1.789864, 102.9994, 102.2249, 102.852, 102.9995, 102.4926, 103.0827, 5.610787, 2.701479, 5.748678e-06, 183358.4, 0.0, 24.56658, 4.990891e-06], [100.0, 100.1194, 24.40213, 100.0, 100.1016, 0.03560248, 158.0093, 1.789864, 99.99963, 99.21942, 99.86005, 99.99973, 99.49659, 100.1016, 5.418124, 2.579388, 5.193695e-06, 183898.6, 0.0, 24.73305, 4.828259e-06], [97.0, 97.17382, 23.39176, 97.0015, 97.15525, 0.03714027, 157.8955, 1.789864, 96.99884, 96.25454, 96.90598, 96.99946, 96.54095, 97.15525, 5.252876, 2.504921, 5.62191e-06, 184439.7, 0.0, 23.73066, 5.229691e-06], [94.0, 94.20774, 23.22087, 94.0002, 94.18903, 0.0374136, 157.7782, 1.789864, 93.99808, 93.27039, 93.92858, 94.00004, 93.56826, 94.18903, 5.073145, 2.409457, 5.538685e-06, 184984.4, 0.0, 23.61211, 6.687232e-06], [91.0, 91.13359, 22.59694, 91.0003, 91.11917, 0.02883498, 157.6522, 1.550068, 91.0004, 90.31659, 90.91559, 90.9996, 90.54901, 91.11917, 4.827745, 2.285596, 4.255465e-06, 185533.6, 0.0, 21.92768, 5.296259e-06], [88.0, 88.18123, 22.48137, 87.9991, 88.16674, 0.02898322, 157.5325, 1.550068, 87.9996, 87.35154, 87.95371, 87.99927, 87.59355, 88.16674, 4.645815, 2.189353, 4.903361e-06, 186084.2, 0.0, 21.34062, 6.20428e-06], [85.0, 85.24232, 22.00163, 84.9979, 85.22751, 0.02961518, 157.4127, 1.550068, 85.00029, 84.40605, 85.0051, 84.99872, 84.65807, 85.22751, 4.439868, 2.085645, 3.898806e-06, 186641.8, 0.0, 20.03455, 4.048067e-06], [82.0, 82.2906, 20.26436, 82.0003, 82.27452, 0.0321541, 157.2935, 1.550068, 81.99943, 81.3944, 82.04882, 81.99944, 81.65225, 82.27452, 4.366601, 2.069786, 4.384861e-06, 187170.4, 0.0, 19.93068, 5.169709e-06], [79.0, 79.35992, 20.65986, 78.9998, 79.34415, 0.03153857, 157.175, 1.550068, 78.99976, 78.46501, 79.10271, 78.99972, 78.73799, 79.34415, 4.123809, 1.934396, 5.660535e-06, 187707.0, 0.0, 20.24228, 3.521332e-06], [76.0, 76.34799, 18.14755, 76.0001, 76.33453, 0.02692852, 157.0442, 1.342398, 75.9988, 75.52364, 76.14176, 76.00082, 75.74333, 76.33453, 3.879228, 1.836679, 5.277406e-06, 188227.8, 0.0, 18.3202, 4.280038e-06], [73.0, 73.40674, 18.83722, 72.9989, 73.39377, 0.02594261, 156.9286, 1.342398, 72.9991, 72.60294, 73.19315, 72.99918, 72.82951, 73.39377, 3.728216, 1.746902, 4.133453e-06, 188764.6, 0.0, 20.32012, 4.874801e-06], [70.0, 70.45695, 17.51673, 70.0003, 70.443, 0.02789829, 156.8115, 1.342398, 70.00086, 69.67221, 70.23128, 69.99956, 69.91183, 70.443, 3.505012, 1.644658, 3.415282e-06, 189312.8, 0.0, 18.10538, 3.636672e-06], [67.0, 67.51137, 17.06142, 66.9986, 67.49705, 0.0286428, 156.6926, 1.342398, 67.0003, 66.75251, 67.27265, 66.99976, 67.00556, 67.49705, 3.329935, 1.557489, 3.637388e-06, 189850.0, 0.0, 17.81273, 2.997229e-06], [64.0, 64.55299, 16.05667, 63.9994, 64.53777, 0.03043512, 156.572, 1.342398, 63.99965, 63.82388, 64.3001, 64.00019, 64.09199, 64.53777, 3.155975, 1.477454, 3.836114e-06, 190372.4, 0.0, 16.65761, 3.137167e-06], [61.0, 61.59684, 15.15327, 61.0012, 61.58071, 0.03224959, 156.4552, 1.342398, 61.00003, 60.89696, 61.32582, 60.99921, 61.18411, 61.58071, 2.932403, 1.370073, 2.715446e-06, 190890.4, 0.0, 15.46223, 4.794554e-06], [58.0, 58.6279, 14.0184, 58.0008, 58.61047, 0.03486038, 156.3434, 1.342398, 57.99915, 57.96364, 58.33762, 57.99934, 58.27135, 58.61047, 2.745862, 1.284894, 2.94282e-06, 191408.4, 0.0, 14.4151, 4.772166e-06], [55.0, 55.65962, 12.33515, 55.0029, 55.63981, 0.03961743, 156.2312, 1.342398, 54.99762, 55.02696, 55.34105, 55.0008, 55.36534, 55.63981, 2.519189, 1.185287, 3.164869e-06, 191919.5, 0.0, 12.86659, 1.828514e-06], [52.0, 52.69421, 11.21244, 51.999, 52.67242, 0.04358434, 156.12, 1.342398, 51.99888, 52.0955, 52.34609, 51.99949, 52.46542, 52.67242, 2.286444, 1.075562, 2.081657e-06, 192439.7, 0.0, 11.76603, 2.789106e-06], [49.0, 49.61418, 9.645293, 49.001, 49.59518, 0.03799937, 156.0042, 1.162551, 48.99919, 49.13845, 49.32293, 49.00038, 49.4487, 49.59518, 2.049105, 0.9693383, 2.419945e-06, 192925.6, 0.0, 10.21014, 2.551699e-06], [46.0, 46.64398, 8.849838, 46.0014, 46.62327, 0.04141489, 155.8991, 1.162551, 45.99971, 46.20159, 46.31906, 45.99925, 46.54721, 46.62327, 1.829977, 0.8624549, 2.062263e-06, 193484.8, 0.0, 8.642792, 8.766135e-07], [43.0, 43.63805, 8.111564, 43.0, 43.61546, 0.04518427, 155.7963, 1.162551, 43.00087, 43.23263, 43.28277, 42.99939, 43.6105, 43.61546, 1.669476, 0.7863123, 2.202847e-06, 194031.9, 0.0, 8.304894, 2.187056e-06], [40.0, 40.60721, 7.850611, 39.9976, 40.58387, 0.04668618, 155.6928, 1.162551, 39.99903, 40.24392, 40.22946, 39.99922, 40.64502, 40.58387, 1.579687, 0.7417823, 1.934699e-06, 194511.3, 0.0, 7.823251, 1.052641e-06], [37.0, 37.55588, 7.570818, 37.0021, 37.53168, 0.04841156, 155.5887, 1.162551, 36.99997, 37.23081, 37.15568, 36.99985, 37.65521, 37.53168, 1.491856, 0.6986331, 1.616464e-06, 195029.6, 0.0, 7.701154, 1.426829e-06], [34.0, 34.39013, 7.129456, 34.002, 34.37085, 0.03855642, 155.4653, 1.006799, 34.00288, 34.19961, 34.07078, 33.99971, 34.53824, 34.37085, 1.389701, 0.6498903, 1.456064e-06, 195501.9, 0.0, 7.197325, 1.830936e-06], [31.0, 31.3295, 6.959681, 30.9971, 31.30975, 0.03949697, 155.3693, 1.006799, 31.00027, 31.15947, 30.98673, 30.99905, 31.52198, 31.30975, 1.305866, 0.6077944, 1.746532e-06, 195974.6, 0.0, 6.855044, 1.3535e-07], [28.0, 28.257, 6.444445, 28.0083, 28.23568, 0.04265477, 155.2754, 1.006799, 27.99751, 28.08427, 27.88122, 28.00025, 28.48138, 28.23568, 1.20443, 0.5603139, 1.207888e-06, 196438.7, 0.0, 6.465166, 2.29124e-06], [25.0, 25.1858, 5.908139, 25.0055, 25.16253, 0.04652672, 155.1906, 1.006799, 25.00147, 24.99086, 24.77406, 24.99832, 25.42586, 25.16253, 1.084087, 0.5032175, 9.614257e-07, 196931.6, 0.0, 5.92471, -5.51895e-08], [22.0, 22.16916, 5.305623, 21.9854, 22.14325, 0.05181037, 155.1142, 1.006799, 22.00671, 21.91764, 21.70696, 21.99982, 22.40575, 22.14325, 0.959603, 0.4446781, 7.916026e-07, 197380.4, 0.0, 5.277611, 2.768679e-07], [19.0, 19.30572, 4.637635, 18.9844, 19.27608, 0.05927295, 155.0499, 1.006799, 18.99661, 18.95241, 18.76765, 19.00061, 19.52011, 19.27608, 0.8426237, 0.390679, 5.587576e-07, 197860.4, 0.0, 4.670142, -7.621961e-08], [16.0, 16.50024, 3.972702, 16.0034, 16.46565, 0.06919378, 154.9962, 1.006799, 15.99681, 16.00464, 15.86607, 15.99389, 16.67341, 16.46565, 0.7071578, 0.3270905, 3.955843e-07, 198345.2, 0.0, 3.981336, -9.093087e-09], [13.0, 13.71888, 3.255681, 13.0265, 13.67666, 0.08443282, 154.9529, 1.006799, 12.99021, 12.98951, 12.9155, 12.99523, 13.83511, 13.67666, 0.5650661, 0.2606204, 4.899574e-08, 199058.5, 0.0, 3.267024, -3.089664e-07], [10.0, 11.02144, 2.634719, 9.9178, 10.96927, 0.1043323, 154.9244, 1.006799, 9.979209, 9.944225, 9.937939, 9.981572, 11.07989, 10.96927, 0.4191188, 0.1915213, 3.509129e-08, 199788.6, 0.0, 2.637912, 3.892924e-07], [7.0, 8.207977, 2.280254, 7.0263, 8.162771, 0.09041306, 154.877, 0.8719131, 6.996675, 6.899136, 6.944581, 6.995916, 8.207738, 8.162771, 0.272072, 0.1212537, 1.590448e-07, 200474.8, 0.0, 2.226699, -2.06841e-07], [4.0, 6.17061, 6.914511, 3.9852, 6.155702, 0.02981624, 154.8519, 0.8719131, 4.007358, 3.946248, 3.912001, 4.007225, 6.219766, 6.155702, 0.1566822, 0.06587024, 3.496313e-07, 201190.7, 0.0, 6.388795, -3.268214e-08], [2.0, 3.439481, -0.8426919, 2.2818, 3.470062, -0.06116255, 154.8119, 0.4359565, 2.275721, 2.314741, 2.136495, 2.275818, 3.587147, 3.470062, 0.06999886, 0.02771, -3.623877e-09, 201712.2, 0.0, -0.8426919, -3.623877e-09]]}])   [LabVIEW 2025]
uses:
  <vilib>/Analysis/6fits.llb/General Linear Fit Algorithm.ctl
  <vilib>/Analysis/NI_AALPro.lvlib
  <vilib>/Analysis/NI_AALBase.lvlib
panel:
  out "processing":i32
  in  "algorithm":T1 items=["SVD", "Givens", "Givens2", "Householder", "LU Decomposition", "Cholesky", "SVD for Rank Deficient H"]
  in  "smooth factor":i32=121
  in  "iteration Number":i32=2
  in  "polynomial order":i32=2
  in  "filtering range":dbl
  in  "limit 2":dbl=0.0005 format="%.3e"
  in  "limit 1":dbl=0.0005 format="%.3e"
  out "note":string
  in  "menu":T2(ring)
  out "comparative":dbl
  in  "start processing":bool
  in  "column to be modified":u16=4
  # "(1) A selected column will be modified by a pre-defined subVI (modify-column_subvi.vi)\n(2) The modified column will replace the original column."
  # "Caution: All rows will be affected."
  # "(1) Select datasets to be processed"
  # "(Not the coulm of the plot but of the original dataset)"
  # "(2) Sort"
  # "i) Sort ?"
  # "ii) Ascending or descendingwhich order?"
  # "descending"
  # "(3)"
  # "(4) Start processing"
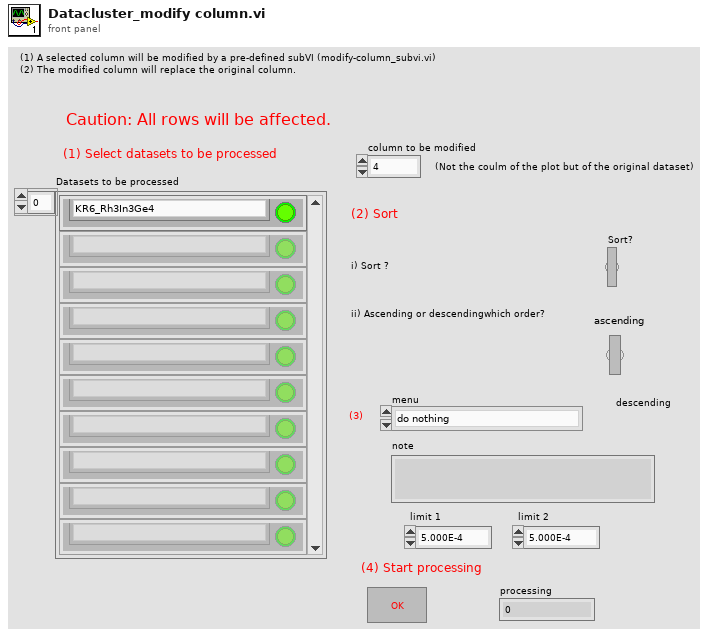
[diagram p1: front panel]
types:
  T1 = typedef "NI_AALPro.lvlib/General Linear Fit Algorithm.ctl" = u16
  T2 = enum16{"do nothing", "remove duplicates", "filtering out of the range", "remove glitches (poly. filter)", "remove glitches (boxcar. filter)", "smoothing only"}
  T3 = cluster{"String":string, "Boolean":bool, "begin":u32, "length":u32, "y weight":dbl}[]
  T4 = enum16{"do nothing", "remove duplicates", "filtering out of the range"}
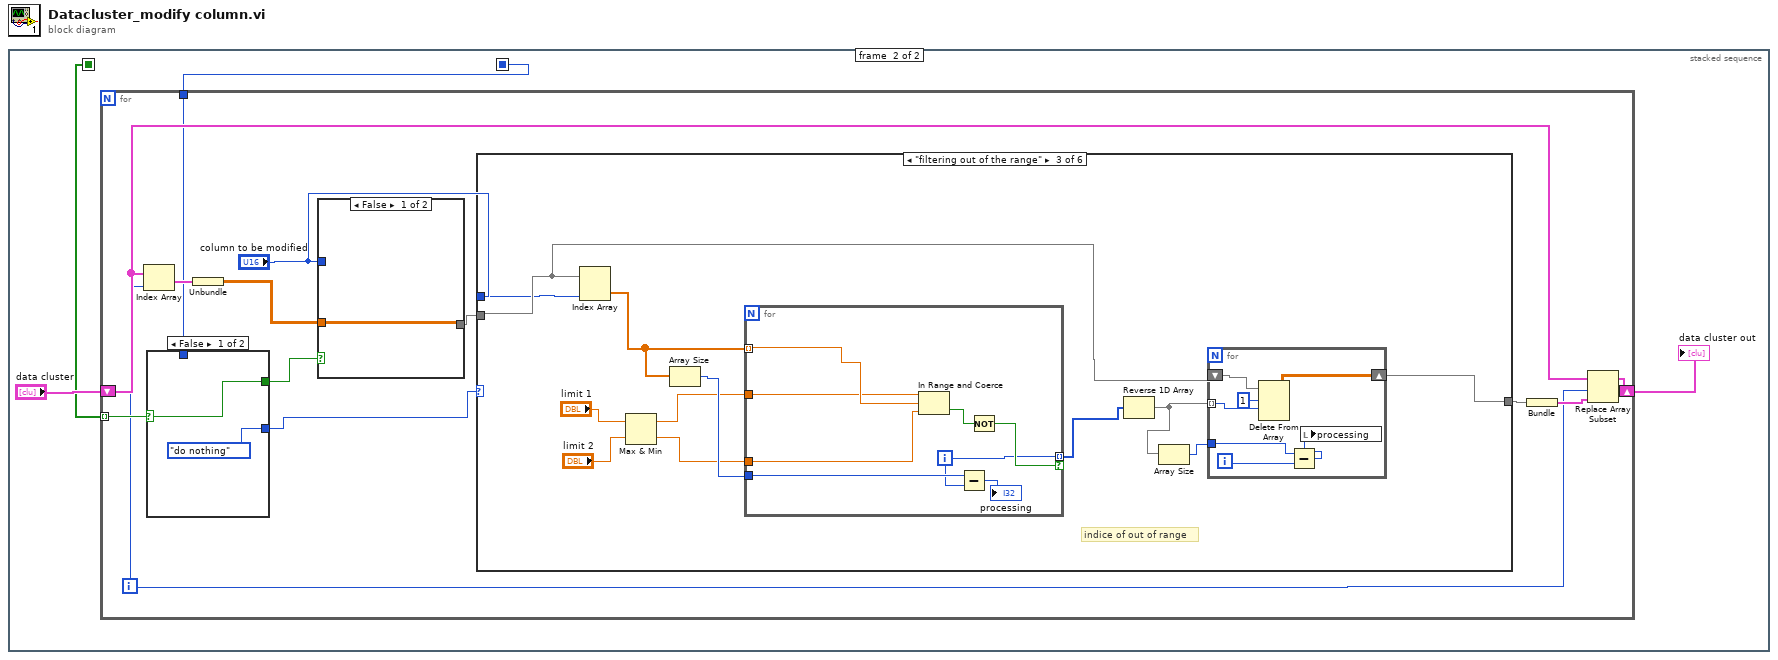
[diagram p0: block diagram]
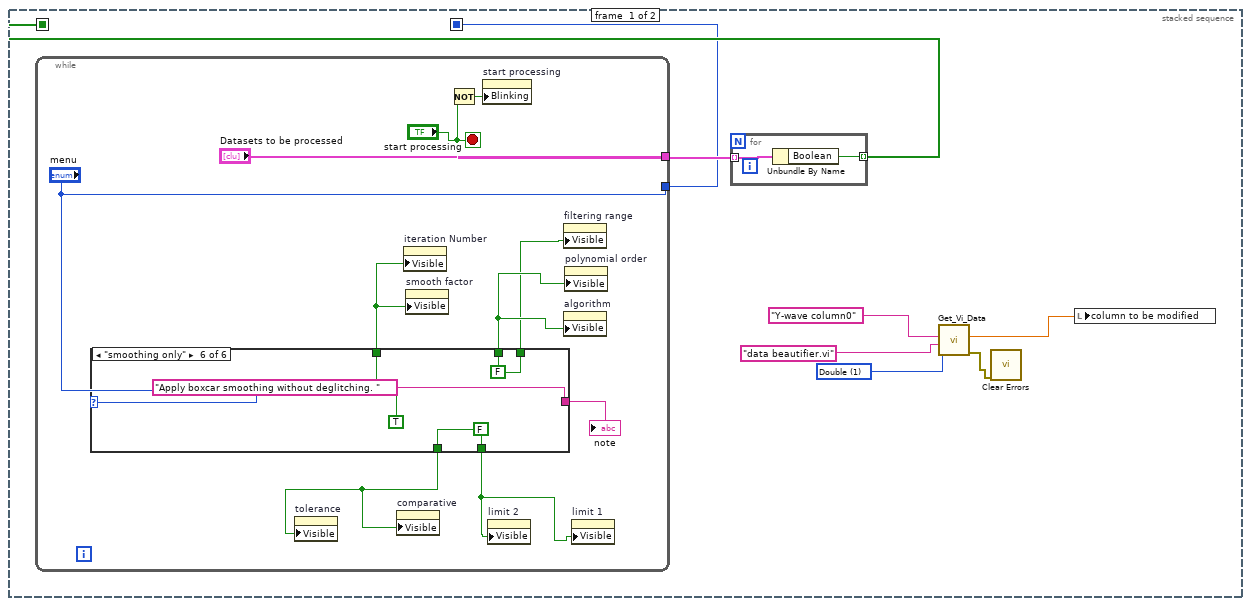
[diagram p2: hidden frame]
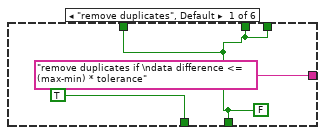
[diagram p3: hidden frame]
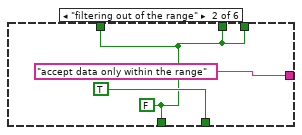
[diagram p4: hidden frame]
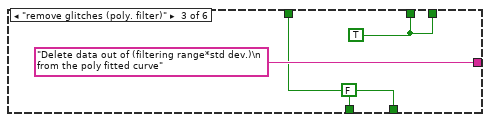
[diagram p5: hidden frame]
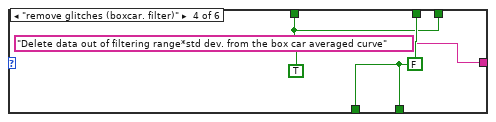
[diagram p6: hidden frame]
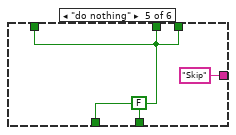
[diagram p7: hidden frame]
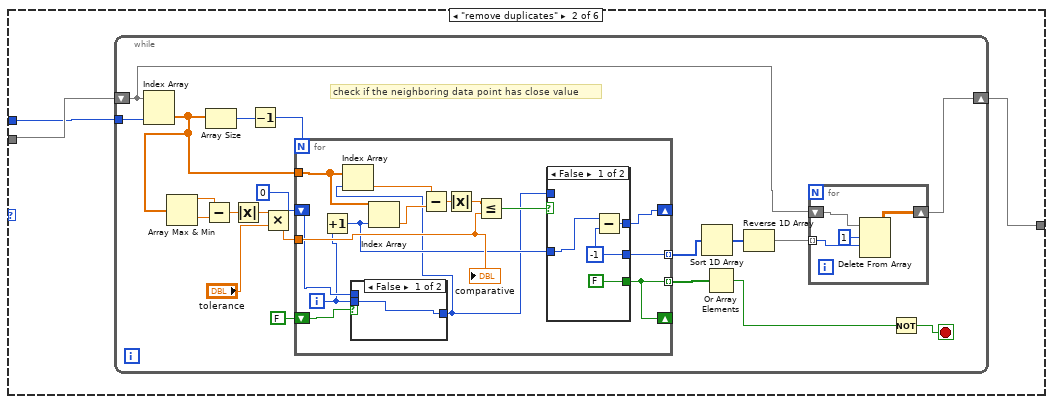
[diagram p9: hidden frame]
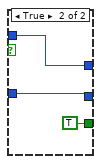
[diagram p11: hidden frame]
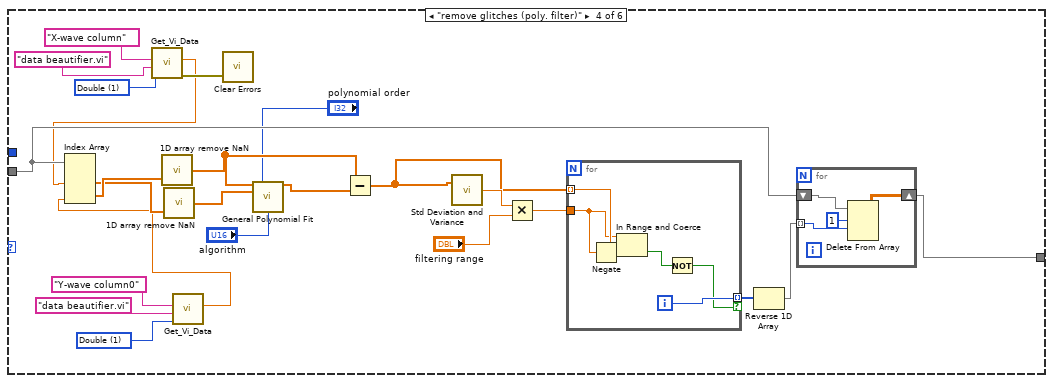
[diagram p12: hidden frame]
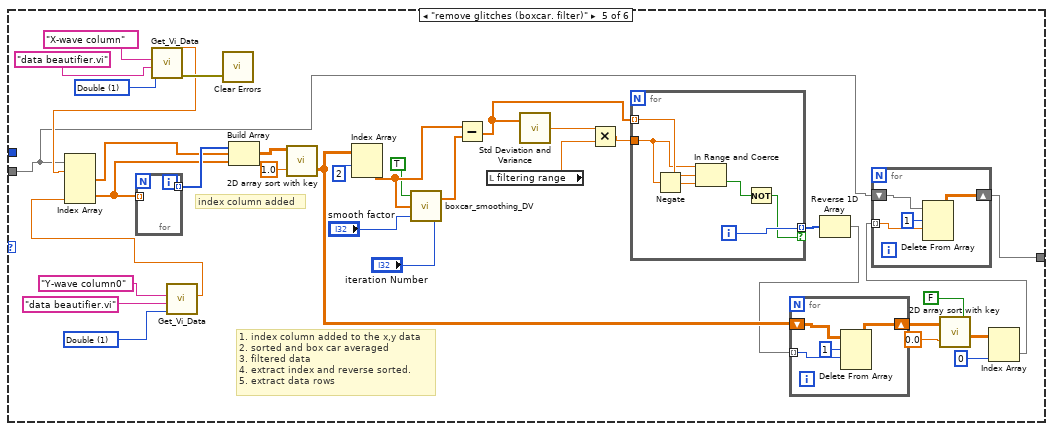
[diagram p13: hidden frame]
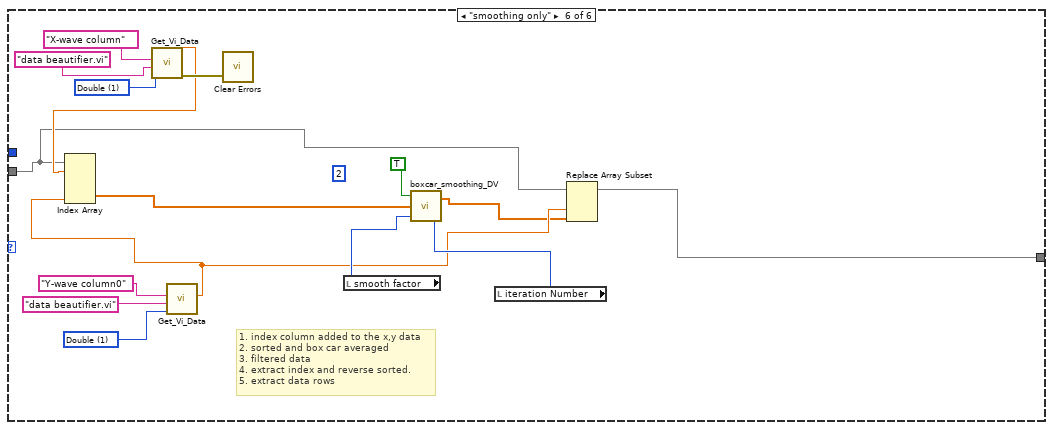
[diagram p14: hidden frame]
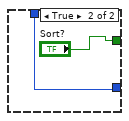
[diagram p15: hidden frame]
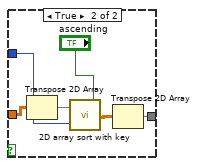
[diagram p16: hidden frame]
diagram:
  n1 = stacked-sequence {
    seq-local: [w7 _] -> [_ w40]
    seq-local: [w6 _] -> [_ w39]
    frame #0 {
      w3 = u16 1 items=["String", "Double", "Boolean", "Variant"] ("Data Type")
      n2 = while {
        tunnel: ["Datasets to be processed"] -> w8
        tunnel: ["menu"] -> w6
        stop <- "start processing" stop-if-true
        n3 = case shown="\"smoothing only\"" "menu" {
          tunnel: ["remove duplicates if \ndata difference <= (max-min) * tolerance" "accept data only within the range" "Delete data out of (filtering range*std dev.)\n from the poly fitted curve" "Delete data out of filtering range*std dev. from the box car averaged curve" "Skip" "Apply boxcar smoothing without deglitching. "] -> w16
          tunnel: [TRUE w24 w28 w32 w33 w36] -> w15
          tunnel: [w21 TRUE w28 w32 w33 w36] -> w14
          tunnel: [w21 w24 w27 w32 w33 w35] -> w13
          tunnel: [w21 w24 w28 w30 w33 TRUE] -> w12
          tunnel: [w21 w24 w27 w30 w33 w35] -> w11
          frame "remove duplicates", Default {
            w21 = FALSE
          }
          frame "filtering out of the range" {
            w24 = FALSE
          }
          frame "remove glitches (poly. filter)" {
            w28 = FALSE
            w27 = TRUE
          }
          frame "remove glitches (boxcar. filter)" {
            w30 = TRUE
            w32 = FALSE
          }
          frame "do nothing" {
            w33 = FALSE
          }
          frame "smoothing only" {
            w36 = FALSE
            w35 = FALSE
          }
        }
        "note" <- w16
        n4 = property on="tolerance" class="DigNum (strict)"("Visible"=w15) -> ()  [unwired: 2 in, 2 out]
        n5 = property on="comparative" class="DigNum (strict)"("Visible"=w15) -> ()  [unwired: 2 in, 2 out]
        n6 = property on="iteration Number" class="DigNum (strict)"("Visible"=w12) -> ()  [unwired: 2 in, 2 out]
        n7 = property on="smooth factor" class="DigNum (strict)"("Visible"=w12) -> ()  [unwired: 2 in, 2 out]
        n8 = Not(x="start processing") -> (.not. x?=w19:bool)
        n9 = property on="start processing" class="Bool"("Blinking"=w19) -> ()  [unwired: 2 in, 2 out]
        n10 = property on="limit 2" class="DigNum (strict)"("Visible"=w14) -> ()  [unwired: 2 in, 2 out]
        n11 = property on="filtering range" class="DigNum (strict)"("Visible"=w11) -> ()  [unwired: 2 in, 2 out]
        n12 = property on="algorithm" class="Ring (strict)"("Visible"=w13) -> ()  [unwired: 2 in, 2 out]
        n13 = property on="polynomial order" class="DigNum (strict)"("Visible"=w13) -> ()  [unwired: 2 in, 2 out]
        n14 = property on="limit 1" class="DigNum (strict)"("Visible"=w14) -> ()  [unwired: 2 in, 2 out]
      }
      n15 = for {
        tunnel: w8 -> [w10] mode=indexing
        tunnel: [w9] -> w7 mode=indexing
        n16 = Unbundle By Name(w10) -> ("Boolean"=w9:bool)
      }
      n17 = call "Get_Vi_Data.vi"("Data Type"=w3, "VI name"="data beautifier.vi", "Control Name"="Y-wave column0") -> ("error out"=w1:errorcluster, "Data (Double)"=w2:dbl)  [unwired: 4 in, 3 out]
      n18 = call <vilib>:"Clear Errors.vi"("error in (no error)"=w1) -> ()  [unwired: 5 in, 2 out]
      n19 = local write "column to be modified"(w2) -> ()
    }
    frame #1 {
      n20 = for {
        shift-right: [w48] -> w41
        shift-left: "data cluster" -> [w51]
        tunnel: w40 -> [w47] mode=indexing
        tunnel: w39 -> [w45]
        i -> [w46]
        n21 = Index Array(array=w51, index=w46) -> (element=w54:cluster{"all rows":dbl[][]})
        n22 = case shown="False" w47 {
          selector: w47 -> [w236 _]
          tunnel: [w236 "Sort?"] -> w55
          tunnel: w45 -> [_ w237]
          tunnel: [T4."do nothing" ("menu") w237] -> w44
          frame False {
          }
          frame True {
          }
        }
        n23 = Unbundle(w54) -> ("all rows"=w53:dbl[][])
        n24 = case shown="False" w55 {
          tunnel: [w239 w240] -> w52
          tunnel: w53 -> [w239 w245]
          tunnel: "column to be modified" -> [_ w242]
          frame False {
          }
          frame True {
            n25 = Transpose 2D Array(2D array=w245) -> (transposed array=w241:dbl[][])
            n26 = call "2D array sort with key.vi"("ascending"="ascending", "key row"=w242, "input"=w241) -> ("output"=w244:dbl[][])
            n27 = Transpose 2D Array(2D array=w244) -> (transposed array=w240:dbl[][])
          }
        }
        n28 = case shown="\"filtering out of the range\"" w44 {
          tunnel: [w56 w57 w117 w152 w200 w219] -> w50
          tunnel: w52 -> [w56 w59 w119 w153 w170 w222]
          tunnel: "column to be modified" -> [_ w58 w118 _ _ _]
          frame "do nothing", Default {
          }
          frame "remove duplicates" {
            n29 = while {
              tunnel: w58 -> [w73]
              shift-right: [w64] -> w57
              shift-left: w59 -> [w65]
              stop <- w74 stop-if-true
              # "check if the neighboring data point has close value"
              n30 = Index Array(array=w65, index (col)=w73) -> (element=w68:dbl[])  [unwired: 1 in]
              n31 = Array Max & Min(array=w68) -> (max value=w67:dbl, min value=w69:dbl)  [unwired: 2 out]
              n32 = Subtract(x=w67, y=w69) -> (x-y=w70:dbl)
              n33 = Array Size(array=w68) -> (size(s)=w63:i32)
              n34 = Absolute Value(x=w70) -> (abs(x)=w72:dbl)
              n35 = Decrement(x=w63) -> (x-1=w62:i32)
              n36 = Multiply(x=w72, y="tolerance") -> (x*y=w66:dbl)
              n37 = for {
                N: w62 -> [_]
                tunnel: w68 -> [w98]
                tunnel: w66 -> [w94]
                tunnel: [w89] -> w78 mode=indexing
                tunnel: [w90] -> w76 mode=indexing
                shift-right: [w88] -> _
                shift-left: 0 -> [w86]
                shift-right: [w90] -> _
                shift-left: FALSE -> [w87]
                i -> [w84]
                n38 = Increment(x=w84) -> (x+1=w92:i32)
                n39 = case shown="False" w87 {
                  tunnel: [w99 w100] -> w85
                  tunnel: w86 -> [_ w100]
                  tunnel: w84 -> [w99 _]
                  frame False {
                  }
                  frame True {
                  }
                }
                n40 = Index Array(array=w98, index=w85) -> (element=w96:dbl)
                n41 = Index Array(array=w98, index=w92) -> (element=w97:dbl)
                n42 = Subtract(x=w96, y=w97) -> (x-y=w95:dbl)
                n43 = Absolute Value(x=w95) -> (abs(x)=w91:dbl)
                n44 = Less Or Equal?(x=w91, y=w94) -> (x <= y?=w93:bool)
                n45 = case shown="False" w93 {
                  tunnel: w92 -> [w102 w107]
                  tunnel: [w103 w107] -> w89
                  tunnel: [FALSE TRUE] -> w90
                  tunnel: [w101 w105] -> w88
                  tunnel: w85 -> [_ w105]
                  frame False {
                    w103 = -1
                    n46 = Subtract(x=w102, y=w103) -> (x-y=w101:i32)
                  }
                  frame True {
                  }
                }
                "comparative" <- w94
              }
              n47 = Sort 1D Array(array=w78) -> (sorted array=w79:i32[])
              n48 = Or Array Elements(Boolean array=w76) -> (logical OR=w75:bool)
              n49 = Reverse 1D Array(array=w79) -> (reversed array=w77:i32[])
              n50 = for {
                tunnel: w77 -> [w82] mode=indexing
                shift-right: [w80] -> w64
                shift-left: w65 -> [w81]
                n51 = Delete From Array(array=w81, length=1, index (row)=w82) -> (array with subset deleted=w80:dbl[][])  [unwired: 1 in, 1 out]
              }
              n52 = Not(x=w75) -> (.not. x?=w74:bool)
            }
          }
          frame "filtering out of the range" {
            # "indice of out of range"
            n53 = Index Array(array=w119, index (col)=w118) -> (element=w115:dbl[])  [unwired: 1 in]
            n54 = Max & Min(x="limit 1", y="limit 2") -> (max(x,y)=w110:dbl, min(x,y)=w108:dbl)
            n55 = Array Size(array=w115) -> (size(s)=w114:i32)
            n56 = for {
              tunnel: w115 -> [w132] mode=indexing
              tunnel: [w130] -> w116 mode=indexing if=w133
              tunnel: w114 -> [w131]
              tunnel: w110 -> [w128]
              tunnel: w108 -> [w127]
              i -> [w130]
              n57 = In Range and Coerce(upper limit=w128, x=w132, lower limit=w127) -> (In Range?=w134:bool)  [unwired: 1 out]
              n58 = Subtract(x=w131, y=w130) -> (x-y=→"processing":i32)
              n59 = Not(x=w134) -> (.not. x?=w133:bool)
            }
            n60 = Reverse 1D Array(array=w116) -> (reversed array=w113:i32[])
            n61 = Array Size(array=w113) -> (size(s)=w112:i32)
            n62 = for {
              tunnel: w113 -> [w125] mode=indexing
              shift-right: [w123] -> w117
              shift-left: w119 -> [w124]
              tunnel: w112 -> [w122]
              i -> [w121]
              n63 = Delete From Array(array=w124, length=1, index (row)=w125) -> (array with subset deleted=w123:dbl[][])  [unwired: 1 in, 1 out]
              n64 = Subtract(x=w122, y=w121) -> (x-y=w120:i32)
              n65 = local write "processing"(w120) -> ()
            }
          }
          frame "remove glitches (poly. filter)" {
            w137 = u16 1 items=["String", "Double", "Boolean", "Variant"] ("Data Type")
            w149 = u16 1 items=["String", "Double", "Boolean", "Variant"] ("Data Type")
            n66 = call "Get_Vi_Data.vi"("Data Type"=w149, "VI name"="data beautifier.vi", "Control Name"="X-wave column") -> ("error out"=w148:errorcluster, "Data (Double)"=w146:dbl)  [unwired: 4 in, 3 out]
            n67 = call "Get_Vi_Data.vi"("Data Type"=w137, "VI name"="data beautifier.vi", "Control Name"="Y-wave column0") -> ("Data (Double)"=w135:dbl)  [unwired: 4 in, 4 out]
            n68 = Index Array(array=w153, index (col) #1=w146, index (col) #2=w135) -> (element #1=w143:dbl[], element #2=w145:dbl[])  [unwired: 2 in]
            n69 = call "1D array remove NaN.vi"("Array input"=w145) -> ("cleaned array"=w144:dbl[])  [unwired: 1 in]
            n70 = call "1D array remove NaN.vi"("Array input"=w143) -> ("cleaned array"=w140:dbl[])  [unwired: 1 in]
            n71 = call <vilib>:"Clear Errors.vi"("error in (no error)"=w148) -> ()  [unwired: 5 in, 2 out]
            n72 = call <vilib>:"General Polynomial Fit.vi"("Y"=w144, "polynomial order"="polynomial order", "X"=w140, "algorithm"="algorithm") -> ("Best Polynomial Fit"=w141:dbl[])  [unwired: 8 in, 3 out]
            n73 = Subtract(x=w144, y=w141) -> (x-y=w147:dbl[])
            n74 = call <vilib>:"Std Deviation and Variance.vi"("X"=w147) -> ("standard deviation"=w158:dbl)  [unwired: 1 in, 2 out]
            n75 = Multiply(x=w158, y="filtering range") -> (x*y=w156:dbl)
            n76 = for {
              tunnel: w147 -> [w165] mode=indexing
              tunnel: [w168] -> w154 mode=indexing if=w166
              tunnel: w156 -> [w164]
              i -> [w168]
              n77 = Negate(x=w164) -> (-x=w163:dbl)
              n78 = In Range and Coerce(upper limit=w164, x=w165, lower limit=w163) -> (In Range?=w167:bool)  [unwired: 1 out]
              n79 = Not(x=w167) -> (.not. x?=w166:bool)
            }
            n80 = Reverse 1D Array(array=w154) -> (reversed array=w155:i32[])
            n81 = for {
              tunnel: w155 -> [w161] mode=indexing
              shift-right: [w159] -> w152
              shift-left: w153 -> [w160]
              n82 = Delete From Array(array=w160, length=1, index (row)=w161) -> (array with subset deleted=w159:dbl[][])  [unwired: 1 in, 1 out]
            }
          }
          frame "remove glitches (boxcar. filter)" {
            w180 = u16 1 items=["String", "Double", "Boolean", "Variant"] ("Data Type")
            w197 = u16 1 items=["String", "Double", "Boolean", "Variant"] ("Data Type")
            # "1. index column added to the x,y data\n2. sorted and box car averaged\n3. filtered data\n4. extract index and reverse sorted.\n5. extract data rows"
            # "index column added"
            n83 = call "Get_Vi_Data.vi"("Data Type"=w197, "VI name"="data beautifier.vi", "Control Name"="X-wave column") -> ("error out"=w196:errorcluster, "Data (Double)"=w189:dbl)  [unwired: 4 in, 3 out]
            n84 = call "Get_Vi_Data.vi"("Data Type"=w180, "VI name"="data beautifier.vi", "Control Name"="Y-wave column0") -> ("Data (Double)"=w178:dbl)  [unwired: 4 in, 4 out]
            n85 = Index Array(array=w170, index (col) #1=w189, index (col) #2=w178) -> (element #1=w187:dbl[], element #2=w188:dbl[])  [unwired: 2 in]
            n86 = for {
              tunnel: w188 -> [_] mode=indexing
              tunnel: [w208] -> w195 mode=indexing
              i -> [w208]
            }
            n87 = call <vilib>:"Clear Errors.vi"("error in (no error)"=w196) -> ()  [unwired: 5 in, 2 out]
            n88 = Build Array(w195, w187, w188) -> (w194:dbl[][])
            n89 = call "2D array sort with key.vi"("key row"=1.0, "input"=w194) -> ("output"=w177:dbl[][])  [unwired: 1 in]
            n90 = Index Array(array=w177, index (row)=2 ("disabled index (col)")) -> (element=w185:dbl[])  [unwired: 1 in]
            n91 = call "boxcar_smoothing_DV.vi"("iteration Number"="iteration Number", "smooth factor"="smooth factor", "raw data"=w185, "NaN filter"=TRUE) -> ("smoothed"=w186:dbl[])
            n92 = Subtract(x=w185, y=w186) -> (x-y=w184:dbl[])
            n93 = local read "filtering range"() -> (w183:dbl)
            n94 = call <vilib>:"Std Deviation and Variance.vi"("X"=w184) -> ("standard deviation"=w203:dbl)  [unwired: 1 in, 2 out]
            n95 = Multiply(x=w203, y=w183) -> (x*y=w202:dbl)
            n96 = for {
              tunnel: w184 -> [w215] mode=indexing
              tunnel: [w218] -> w201 mode=indexing if=w216
              tunnel: w202 -> [w214]
              i -> [w218]
              n97 = Negate(x=w214) -> (-x=w213:dbl)
              n98 = In Range and Coerce(upper limit=w214, x=w215, lower limit=w213) -> (In Range?=w217:bool)  [unwired: 1 out]
              n99 = Not(x=w217) -> (.not. x?=w216:bool)
            }
            n100 = Reverse 1D Array(array=w201) -> (reversed array=w176:i32[])
            n101 = for {
              tunnel: w176 -> [w206] mode=indexing
              shift-right: [w204] -> w175
              shift-left: w177 -> [w205]
              n102 = Delete From Array(array=w205, length=1, index (row)=w206) -> (array with subset deleted=w204:dbl[][])  [unwired: 1 in, 1 out]
            }
            n103 = call "2D array sort with key.vi"("ascending"=FALSE, "key row"=0.0, "input"=w175) -> ("output"=w173:dbl[][])
            n104 = Index Array(array=w173, index (row)=0) -> (element=w171:dbl[])  [unwired: 1 in]
            n105 = for {
              tunnel: w171 -> [w211] mode=indexing
              shift-right: [w209] -> w200
              shift-left: w170 -> [w210]
              n106 = Delete From Array(array=w210, length=1, index (row)=w211) -> (array with subset deleted=w209:dbl[][])  [unwired: 1 in, 1 out]
            }
          }
          frame "smoothing only" {
            w227 = u16 1 items=["String", "Double", "Boolean", "Variant"] ("Data Type")
            (unwired) 2 ("disabled index (col)")
            w232 = u16 1 items=["String", "Double", "Boolean", "Variant"] ("Data Type")
            # "1. index column added to the x,y data\n2. sorted and box car averaged\n3. filtered data\n4. extract index and reverse sorted.\n5. extract data rows"
            n107 = call "Get_Vi_Data.vi"("Data Type"=w232, "VI name"="data beautifier.vi", "Control Name"="X-wave column") -> ("error out"=w231:errorcluster, "Data (Double)"=w230:dbl)  [unwired: 4 in, 3 out]
            n108 = call "Get_Vi_Data.vi"("Data Type"=w227, "VI name"="data beautifier.vi", "Control Name"="Y-wave column0") -> ("Data (Double)"=w221:dbl)  [unwired: 4 in, 4 out]
            n109 = Index Array(array=w222, index (col) #1=w230, index (col) #2=w221) -> (element #2=w223:dbl[])  [unwired: 2 in, 1 out]
            n110 = call <vilib>:"Clear Errors.vi"("error in (no error)"=w231) -> ()  [unwired: 5 in, 2 out]
            n111 = local read "smooth factor"() -> (w225:i32)
            n112 = local read "iteration Number"() -> (w224:i32)
            n113 = call "boxcar_smoothing_DV.vi"("iteration Number"=w224, "smooth factor"=w225, "raw data"=w223, "NaN filter"=TRUE) -> ("smoothed"=w220:dbl[])
            n114 = Replace Array Subset(array=w222, new element=w220, index (col)=w221) -> (w219:dbl[][])  [unwired: 1 in]
          }
        }
        n115 = Bundle("all rows"=w50) -> (w49:cluster{"all rows":dbl[][]})  [unwired: 1 in]
        n116 = Replace Array Subset(array=w51, new element=w49, index=w46) -> (w48:cluster{"all rows":dbl[][]}[])
      }
      "data cluster out" <- w41
    }
  }
